vi "zskk.vi"() -> ()   [LabVIEW 2017]
panel:
  out "y":dbl
  in  "k":dbl
  in  "x":dbl
  in  "b":dbl
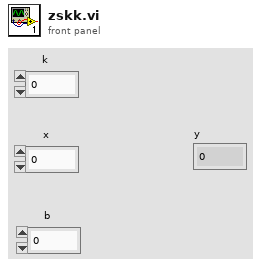
[diagram p1: front panel]
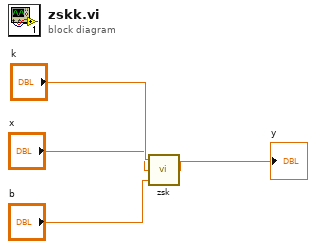
[diagram p0: block diagram]
diagram:
  n1 = call "zsk.vi"("b 3"="b", "x"="x", "k"="k") -> ("数值"=→"y":dbl)
